vi "Bundle FPGA Configuration.vi"(8 "error in (no error)":errorcluster, 11 "FPGA Interface (Old)":T5) -> (0 "error out":errorcluster, 3 "All FPGA Configuration Values":T1)   [LabVIEW 2013]
uses:
  controls/FPGA VI Reference.ctl
  controls/All FPGA Configuration Values.ctl
  controls/FPGA State.ctl
  controls/Raw Values.ctl
  controls/Control Configuration.ctl
  <vilib>/Utility/error.llb/Error Cluster From Error Code.vi
  <vilib>/rvi/errors/niLvFpgaAdjustHostInterfaceError.vi
  <vilib>/rvi/interface/nirviReadWriteControl/nirviReadWriteControl.xnode
  FPGA Bitfiles/crio-FPGA-contro_FPGATarget_FPGAMain_4HKUk4gb9wY.lvbitx
  NiFpgaLv.dll
panel:
  in  "FPGA VI Reference":refnum<k20>
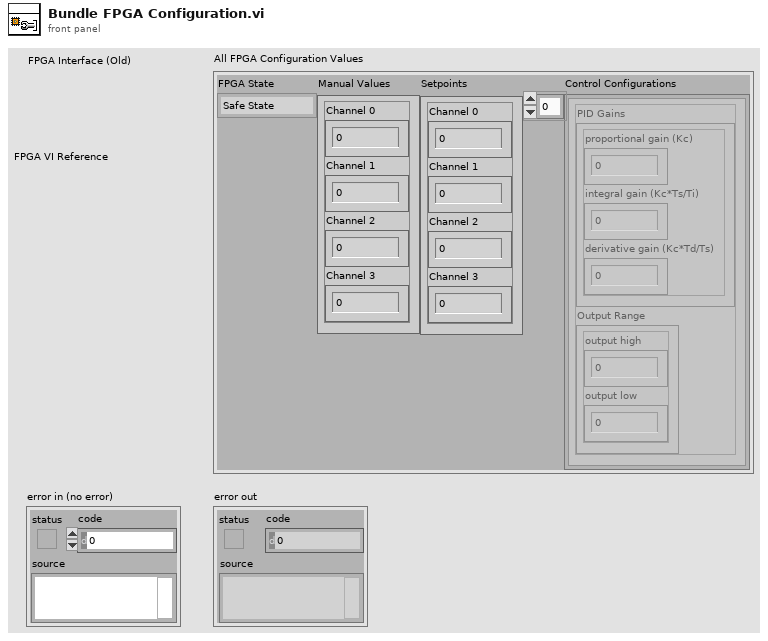
[diagram p1: front panel]
types:
  T1 = typedef "All FPGA Configuration Values.ctl" = cluster{"FPGA State":T2, "Manual Values":T3, "Setpoints":T3, "Control Configurations":T4[]}
  T2 = typedef "FPGA State.ctl" = enum16{"Safe State", "Manual", "Control (PID)"}
  T3 = typedef "Raw Values.ctl" = cluster{"Channel 0":fxp<+/-,20,7>, "Channel 1":fxp<+/-,20,7>, "Channel 2":fxp<+/-,20,7>, "Channel 3":fxp<+/-,20,14>}
  T4 = typedef "Control Configuration.ctl" = cluster{"PID Gains":cluster{"proportional gain (Kc)":fxp<+/-,16,8>, "integral gain (Kc*Ts/Ti)":fxp<+/-,16,8>, "derivative gain (Kc*Td/Ts)":fxp<+/-,16,8>}, "Output Range":cluster{"output high":fxp<+/-,16,7>, "output low":fxp<+/-,16,7>}}
  T5 = typedef "FPGA VI Reference.ctl" = refnum<k20>
  T6 = cluster{"Channel 0 Setpoint (Force)":fxp<+/-,20,7>, "Channel 1 Setpoint  (Position)":fxp<+/-,20,7>, "Channel 2 Setpoint":fxp<+/-,20,7>, "Channel 3 Setpoint":fxp<+/-,16,7>}
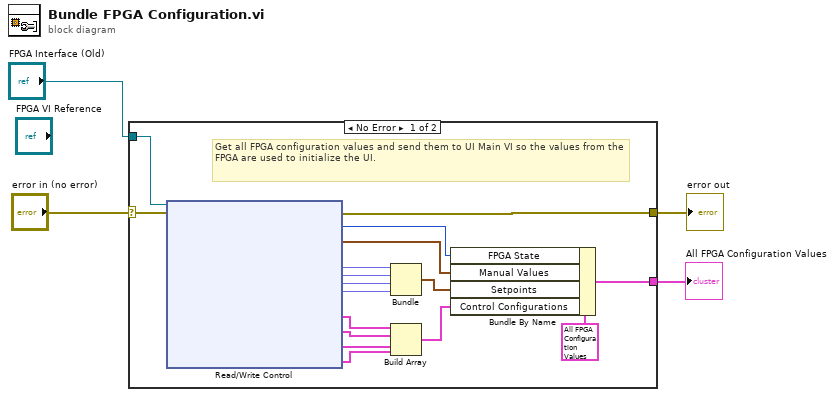
[diagram p0: block diagram]
diagram:
  n1 = case shown="No Error" "error in (no error)" {
    selector: "error in (no error)" -> [w21 w22]
    tunnel: "FPGA Interface (Old)" -> [w20 _]
    tunnel: [w19 w22] -> w3
    tunnel: [w7 _] -> w2
    frame No Error {
      # "Get all FPGA configuration values and send them to UI Main VI so the values from the FPGA are used to initialize the UI."
      n2 = xnode "Read/Write Control"("FPGA VI Reference In"=w20, "error in"=w21) -> ("error out"=w19:errorcluster, "Current FPGA State"=w6:T2, "Manual Values"=w17:T3, "Channel 0 Setpoint (Force)"=w16:fxp<+/-,20,7>, "Channel 1 Setpoint  (Position)"=w15:fxp<+/-,20,7>, "Channel 2 Setpoint"=w14:fxp<+/-,20,7>, "Channel 3 Setpoint"=w13:fxp<+/-,16,7>, "Channel 0 Configuration"=w12:T4, "Channel 1 Configuration"=w11:T4, "Channel 2 Configuration"=w10:T4, "Channel 3 Configuration"=w9:T4)  [unwired: 1 out]
      n3 = Bundle("Channel 0 Setpoint (Force)"=w16, "Channel 1 Setpoint  (Position)"=w15, "Channel 2 Setpoint"=w14, "Channel 3 Setpoint"=w13) -> (w5:T6)  [unwired: 1 in]
      n4 = Build Array(w12, w11, w10, w9) -> (w8:T4[])
      n5 = Bundle By Name(cluster=T1 {"FPGA State"=enum."Safe State", "Manual Values"={"Channel 0"=0.0, "Channel 1"=0.0, "Channel 2"=0.0, "Channel 3"=0.0}, "Setpoints"={"Channel 0"=0.0, "Channel 1"=0.0, "Channel 2"=0.0, "Channel 3"=0.0}, "Control Configurations"=[]} ("All FPGA Configuration Values"), "FPGA State"=w6, "Manual Values"=w17, "Setpoints"=w5, "Control Configurations"=w8) -> (w7:T1)
    }
    frame Error {
    }
  }
  "error out" <- w3
  "All FPGA Configuration Values" <- w2
